vi "connect (SubVI).vi"() -> (0 "error out":errorcluster, 3 "x != 0?":bool)   [LabVIEW 2017]
uses:
  Unicorn Labview Library/Unicorn Library.lvlib
  Global_BOC (SubVI).vi
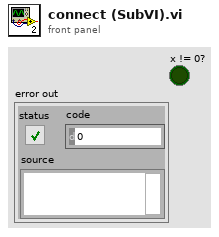
[diagram p1: front panel]
types:
  T1 = typedef "Unicorn Library.lvlib/AnswerUDP.ctl" = cluster{"IP":string, "Port":u16, "DataVersion":u16, "ModbusAddress":i32, "type_version":string, "Description":string, "Serial":string, "ServerPort":u16}
  T2 = typedef "paramUnicorn.ctl" = cluster{"conParam":T3, "Param":T4}
  T3 = typedef "Unicorn Library.lvlib/connectionParam.ctl" = cluster{"ReadIntParam":bool, "ReadDescrParam":bool, "ReadFloatParam":bool, "debug":bool, "ReadJSON":bool, "IP_address":string, "N_attempts":i32, "type_con":enum16{"Serial", "TCP"}, "MB_address":i32, "VISA":refnum<visa-resource-name>, "connection ID":refnum<k5>, "nameDevices":string, "timeout":i32, "port":u16, "type_version":string, "baud_rate":u32, "VersionControl":bool, "TCP_conn":bool}
  T4 = typedef "Unicorn Library.lvlib/JSONParam.ctl" = cluster{"ParamInt":string[][], "ParamTelemetry":string[][], "ParamFloat":string[][], "TableCount":i32[][], "NeedParamPrepare":bool[], "NumParam":cluster{"NTelem":i32, "NInt":i32, "NFloat":i32}, "NTable":i32}
  T5 = typedef "Unicorn Library.lvlib/unicorn_Param.ctl" = cluster{"conParam":T6, "Param":T7}
  T6 = typedef "Unicorn Library.lvlib/unicorn_conn.ctl" = cluster{"ReadIntParam":bool, "ReadDescrParam":bool, "ReadFloatParam":bool, "debug":bool, "ReadJSON":bool, "IP_address":string, "N_attempts":i32, "type_con":enum16{"Serial", "TCP"}, "MB_address":i32, "VISA":refnum<visa-resource-name>, "connection ID":refnum<k5>, "nameDevices":string, "timeout":i32, "port":u16, "type_version":string, "baud_rate":u32, "VersionControl":bool, "TCP_conn":bool}
  T7 = typedef "Unicorn Library.lvlib/unicorn_JSON.ctl" = cluster{"NumParam":cluster{"NTelem":i32, "NInt":i32, "NFloat":i32, "NTable":i32}, "ParamInt":T8, "Telemetry":T9, "Table":T10, "ParamFloat":T11}
  T8 = typedef "Unicorn Library.lvlib/unicorn_ParamInt.ctl" = cluster{"ID":string, "Num":i32, "Name":string, "Type":string, "Enum":string, "Desc":string, "Unit":string, "Access":string, "FormatStr":string, "Min":i32, "Max":i32}[]
  T9 = typedef "Unicorn Library.lvlib/unicorn_Telemetry.ctl" = cluster{"ID":string, "Num":i32, "Name":string, "Desc":string, "Unit":string, "FormatStr":string, "Min":i32, "Max":i32}[]
  T10 = typedef "Unicorn Library.lvlib/unicorn_Table.ctl" = cluster{"Num":i32, "Access":string, "ColumnCount":i32, "NeedParamPrepare":bool, "Columns":cluster{"Column":i32, "Desc":string, "Name":string}[], "DataType":string, "FormatStr":string, "ID":string, "Name":string, "RowCount":i32, "Rows":cluster{"Desc":string, "ID":string, "Max":i32, "Min":i32, "Name":string, "Row":i32, "Unit":string}[], "Type":string}[]
  T11 = typedef "Unicorn Library.lvlib/unicorn_ParamFloat.ctl" = cluster{"ID":string, "Num":i32, "Name":string, "Type":string, "Enum":string, "Desc":string, "Unit":string, "Access":string, "FormatStr":string, "Min":i32, "Max":i32}[]
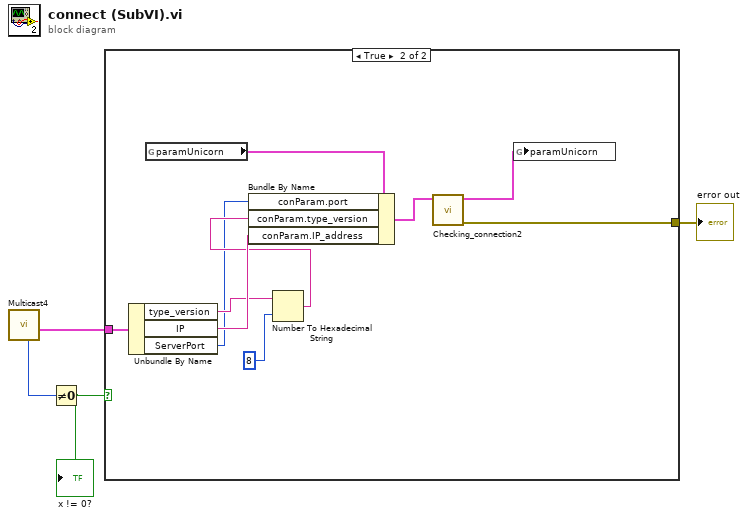
[diagram p0: block diagram]
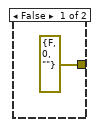
[diagram p2: hidden frame]
diagram:
  n1 = call "Multicast4.vi"() -> ("selDevicesT"=w1:T1, "Sel_IP_hex"=w2:u32)  [unwired: 7 in, 3 out]
  n2 = Not Equal To 0?(x=w2) -> (x != 0?=w3:bool)
  "x != 0?" <- w3
  n3 = case shown="True" w3 {
    tunnel: w1 -> [_ w9]
    tunnel: [errorcluster {"status"=FALSE, "code"=0, "source"=""} ("error out") w8] -> w4
    frame False {
    }
    frame True {
      n4 = Unbundle By Name(w9) -> ("type_version"=w14:string, "IP"=w15:string, "ServerPort"=w11:u16)
      n5 = global read "Global_BOC (SubVI).vi" "paramUnicorn"() -> (w7:T2)
      n6 = Number To Hexadecimal String(1:i16 8 ("width (-)"), 2:w14) -> (0:w12:string)
      n7 = Bundle By Name(cluster=w7, "conParam.port"=w11, "conParam.type_version"=w12, "conParam.IP_address"=w15) -> (w10:T2)
      n8 = call "Checking_connection2.vi"("paramUnicornIn"=w10) -> ("error out"=w8:errorcluster, "paramUnicorn"=w6:T5)  [unwired: 7 in, 2 out]
      n9 = global write "Global_BOC (SubVI).vi" "paramUnicorn"(w6) -> ()
    }
  }
  "error out" <- w4
